vi "Fire Stop Event.vi"(8 "error in (no error)":errorcluster, 11 "Stop Event in":refnum<user-event>) -> (0 "error out":errorcluster)   [LabVIEW 2016, in "Trace Grabber.lvlib"]
uses:
  Trace Grabber.lvlib
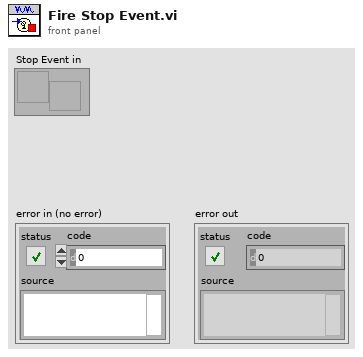
[diagram p1: front panel]
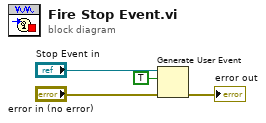
[diagram p0: block diagram]
diagram:
  n1 = Generate User Event(user event="Stop Event in", event data cluster=TRUE ("event data"), error in="error in (no error)") -> (error out=→"error out":errorcluster)  [unwired: 1 in, 1 out]
